vi "zeroHardpointActuatorSteps.vi"(8 "error in (no error)":errorcluster, 11 "Model in":refnum<class "Model.lvclass">) -> (0 "error out":errorcluster, 3 "Model out":refnum<class "Model.lvclass">)   [LabVIEW 2016, in "Model.lvclass"]
uses:
  Model.lvclass
  Model.lvclass/Model.ctl
  ILCCommunications/ILCCommunications.lvclass/ILCCommunications.ctl
  Common_RT_HPILC/HPILC/HPILC.lvclass/HPILC.ctl
  ILCCommunications/getHPs.vi
  ILCCommunications/setHPs.vi
  Common_RT_HPILC/HPILC/getHPData.vi
  Common_RT_HPILC/HPILC/setHPData.vi
  ILCCommunications/ILCCommunications.lvclass
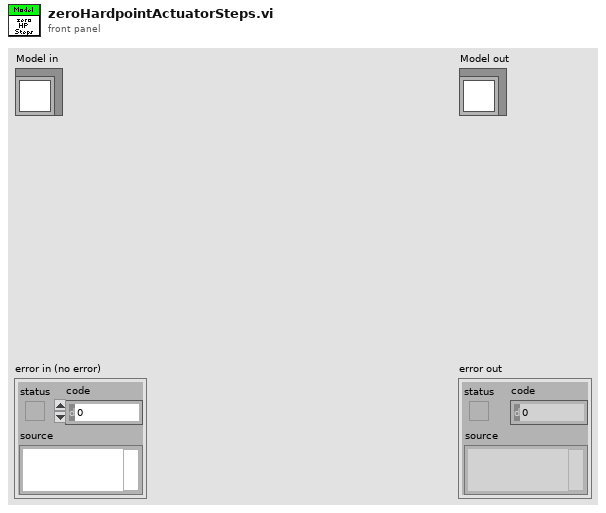
[diagram p1: front panel]
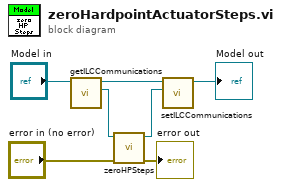
[diagram p0: block diagram]
diagram:
  n1 = call "getILCCommunications.vi"("Model in"="Model in") -> ("ILCCommunications"=w7:refnum<class "ILCCommunications.lvclass">, "Model out"=w5:refnum<class "Model.lvclass">)  [unwired: 9 in]
  n2 = call "zeroHPSteps.vi"("error in (no error)"="error in (no error)", "ILCCommunications in"=w7) -> ("error out"=→"error out":errorcluster, "ILCCommunications out"=w6:refnum<class "ILCCommunications.lvclass">)  [unwired: 8 in]
  n3 = call "setILCCommunications.vi"("ILCCommunications"=w6, "Model in"=w5) -> ("Model out"=→"Model out":refnum<class "Model.lvclass">)  [unwired: 9 in]
